vi "ATF-Pumb DAta to host.vi"(8 "error in (no error)":errorcluster, 11 "Err":refnum<queue>) -> (0 "error out":errorcluster, 3 "data":string)   [LabVIEW 2022 SP3]
uses:
  RT Controls/SeCrTs-Data Type Control screen.ctl
  RT Controls/SeCrTs-FGV Read write.ctl
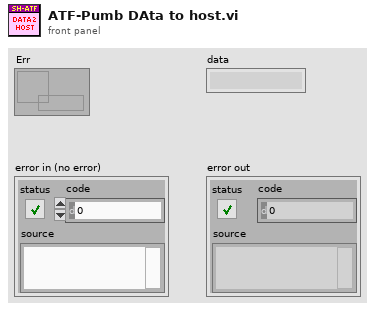
[diagram p1: front panel]
types:
  T1 = typedef "SeCrTs-FGV Read write.ctl" = enum16{"Write", "Read"}
  T2 = typedef "SeCrTs-Data Type Control screen.ctl" = cluster{"DI_Data":digitalwaveform[], "Drive_A_C":waveform(dbl)[], "Drive_A_D":waveform(dbl)[], "Drive_L_C":waveform(dbl)[], "Drive_L_D":waveform(dbl)[], "Loop Status":bool[], "CDT Timer":dbl, "RT Error":cluster{"Error Code":string, "Error Source":string}, "DO":waveform(dbl)[], "SEQ Monitor":string[], "Device List":string}
  T3 = enum16{"Init", "Read 'All'", "Read 'n'", "Read '1'", "Write '1'", "Write 'n'", "Write 'All'"}
  T4 = cluster{"Error Code":string, "Error Source":string}
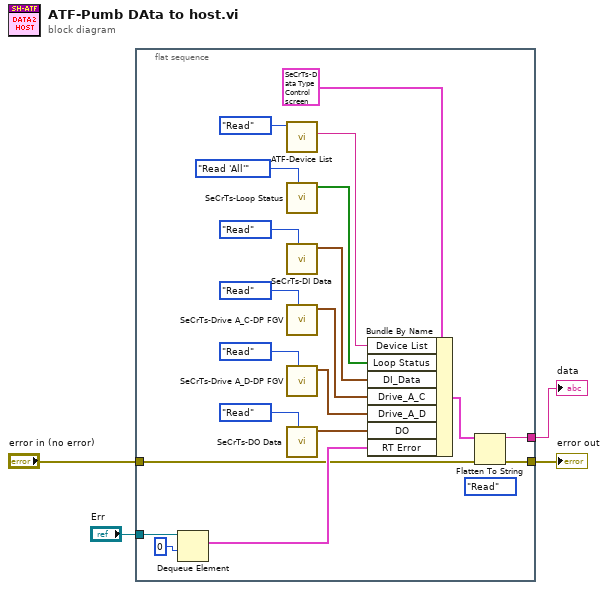
[diagram p0: block diagram]
diagram:
  n1 = flat-sequence {
    tunnel: "error in (no error)" -> [w7]
    tunnel: [w8] -> w3
    tunnel: "Err" -> [w6]
    tunnel: [w5] -> w1
    frame #0 {
      (unwired) enum16{"Write", "Read"}."Read" ("Write/Read")
      n2 = Dequeue Element(queue=w6, timeout in ms (-1)=0) -> (element=w20:T4)  [unwired: 1 in, 3 out]
      n3 = call "ATF-Device List.vi"("Enum"=enum16{"Write", "Read"}."Read") -> ("DL 2"=w10:string)  [unwired: 9 in, 1 out]
      n4 = call "SeCrTs-Loop Status.vi"("Option"=T3."Read 'All'") -> ("Status List Out"=w23:bool[])  [unwired: 8 in, 2 out]
      n5 = call "SeCrTs-DI Data.vi"("Enum"=enum16{"Write", "Read"}."Read") -> ("Out_DI data"=w18:digitalwaveform[])  [unwired: 10 in]
      n6 = call "SeCrTs-Drive A_C-DP FGV.vi"("Write/Read"=SeCrTs-FGV_Read_write."Read") -> ("Drive A_C  data"=w16:waveform(dbl)[])  [unwired: 9 in, 1 out]
      n7 = call "SeCrTs-Drive A_D-DP FGV.vi"("Write/Read"=SeCrTs-FGV_Read_write."Read") -> ("Drive A_D data"=w14:waveform(dbl)[])  [unwired: 9 in, 1 out]
      n8 = call "SeCrTs-DO Data.vi"("Enum"=enum16{"Write", "Read"}."Read") -> ("out_DO data"=w12:waveform(dbl)[])  [unwired: 10 in]
      n9 = Bundle By Name(cluster=T2 {"DI_Data"=[], "Drive_A_C"=[], "Drive_A_D"=[], "Drive_L_C"=[], "Drive_L_D"=[], "Loop Status"=[], "CDT Timer"=0.0, "RT Error"={"Error Code"="", "Error Source"=""}, "DO"=[], "SEQ Monitor"=[], "Device List"=""} ("Cluster"), "Device List"=w10, "Loop Status"=w23, "DI_Data"=w18, "Drive_A_C"=w16, "Drive_A_D"=w14, "DO"=w12, "RT Error"=w20) -> (w9:T2)
      n10 = Flatten To String(anything=w9, error in (no error)=w7) -> (data string=w5:string, error out=w8:errorcluster)  [unwired: 2 in, 1 out]
    }
  }
  "error out" <- w3
  "data" <- w1
